vi "Global_Read_INI_Sub_VI_SM.vi"(0 "Config File Path":path) -> (4 "output cluster":T1)   [LabVIEW 2017]
uses:
  <vilib>/Utility/config.llb/Read Key (U32).vi
  <vilib>/Utility/config.llb/Read Key (String).vi
  <vilib>/Utility/config.llb/Read Key (Path).vi
  <vilib>/Utility/config.llb/NI_LVConfig.lvlib
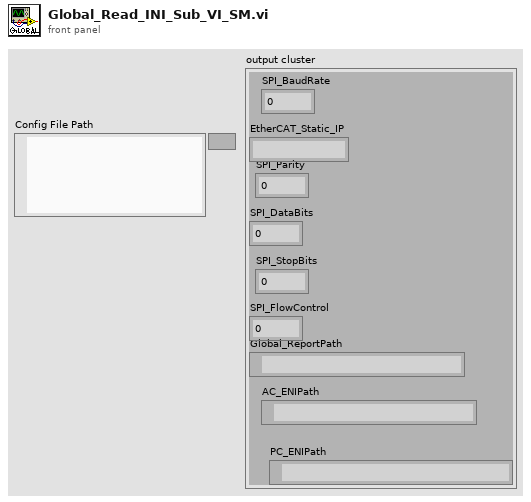
[diagram p1: front panel]
types:
  T1 = cluster{"SPI_BaudRate":u32, "EtherCAT_Static_IP":string, "SPI_Parity":u16, "SPI_DataBits":u16, "SPI_StopBits":u16, "SPI_FlowControl":u16, "Global_ReportPath":path, "AC_ENIPath":path, "PC_ENIPath":path}
  T2 = typedef "NI_LVConfig.lvlib/Config Data RefNum.ctl" = refnum<k1>
  T3 = cluster{u32, "value":string, u16, u16, u16, u16, "value":path, "value":path, "value":path}
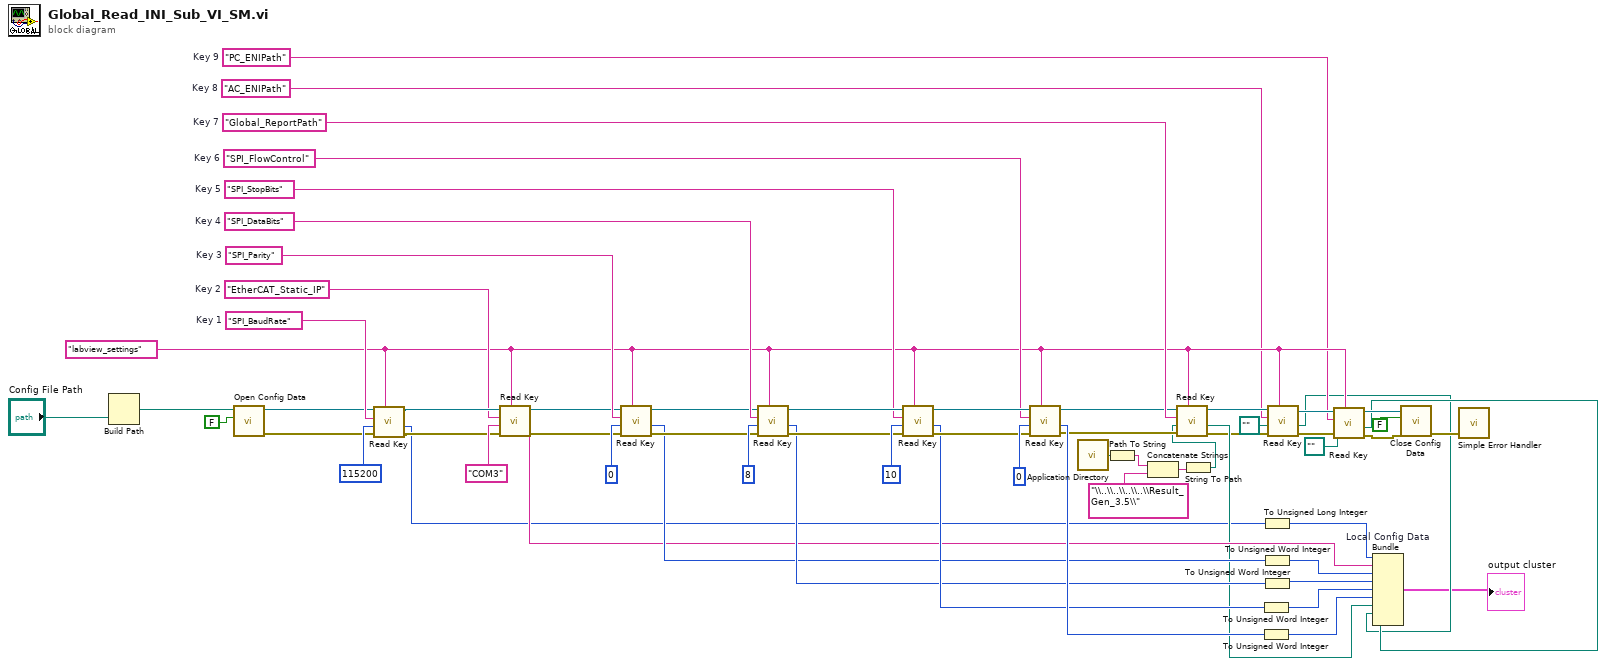
[diagram p0: block diagram]
diagram:
  w6 = "PC_ENIPath"  # Key 9
  w7 = "AC_ENIPath"  # Key 8
  w57 = "Global_ReportPath"  # Key 7
  w53 = "SPI_FlowControl"  # Key 6
  w49 = "SPI_StopBits"  # Key 5
  w47 = "SPI_DataBits"  # Key 4
  w35 = "SPI_Parity"  # Key 3
  w34 = "EtherCAT_Static_IP"  # Key 2
  w40 = "SPI_BaudRate"  # Key 1
  w8 = "labview_settings" ("section")
  n1 = Build Path(name or relative path="Config File Path") -> (appended path=w22:path)  [unwired: 1 in]
  n2 = call <vilib>:"Open Config Data.vi"("create file if necessary (T)"=FALSE ("create file if necessary? (T)"), "configuration file path"=w22) -> ("error out"=w41:errorcluster, "refnum"=w39:T2)  [unwired: 7 in, 1 out]
  n3 = call-poly <vilib>:"Read Key.vi"("section"=w8, "error in (no error)"=w41, "default value"=u32 115200, "key"=w40, "refnum"=w39) -> ("error out"=w42:errorcluster, "value"=w20:u32, "refnum out"=w43:T2)  [unwired: 4 out]
  n4 = call-poly <vilib>:"Read Key.vi"("section"=w8, "error in (no error)"=w42, "default value"="COM3", "key"=w34, "refnum"=w43) -> ("error out"=w33:errorcluster, "value"=w29:string, "refnum out"=w32:T2)  [unwired: 1 in, 3 out]
  n5 = call-poly <vilib>:"Read Key.vi"("section"=w8, "error in (no error)"=w33, "default value"=u32 0, "key"=w35, "refnum"=w32) -> ("error out"=w46:errorcluster, "value"=w44:u32, "refnum out"=w45:T2)  [unwired: 4 out]
  n6 = call-poly <vilib>:"Read Key.vi"("section"=w8, "error in (no error)"=w46, "default value"=u32 8, "key"=w47, "refnum"=w45) -> ("error out"=w51:errorcluster, "value"=w48:u32, "refnum out"=w50:T2)  [unwired: 4 out]
  n7 = call-poly <vilib>:"Read Key.vi"("section"=w8, "error in (no error)"=w51, "default value"=u32 10, "key"=w49, "refnum"=w50) -> ("error out"=w55:errorcluster, "value"=w52:u32, "refnum out"=w54:T2)  [unwired: 4 out]
  n8 = call-poly <vilib>:"Read Key.vi"("section"=w8, "error in (no error)"=w55, "default value"=u32 0, "key"=w53, "refnum"=w54) -> ("error out"=w30:errorcluster, "value"=w56:u32, "refnum out"=w31:T2)  [unwired: 4 out]
  n9 = call <vilib>:"Application Directory.vi"() -> ("Application Directory"=w16:path)
  n10 = Path To String(path=w16) -> (string=w19:string)
  n11 = Concatenate Strings(w19, "\\..\\..\\..\\..\\Result_Gen_3.5\\" ("string")) -> (w17:string)
  n12 = String To Path(string=w17) -> (path=w15:path)
  n13 = call-poly <vilib>:"Read Key.vi"("section"=w8, "error in (no error)"=w30, "default value"=w15, "key"=w57, "refnum"=w31) -> ("error out"=w14:errorcluster, "value"=w24:path, "refnum out"=w13:T2)  [unwired: 1 in, 3 out]
  n14 = To Unsigned Word Integer(number=w52) -> (unsigned 16bit integer=w26:u16)
  n15 = To Unsigned Word Integer(number=w56) -> (unsigned 16bit integer=w25:u16)
  n16 = To Unsigned Long Integer(number=w20) -> (unsigned 32bit integer=w21:u32)
  n17 = To Unsigned Word Integer(number=w44) -> (unsigned 16bit integer=w28:u16)
  n18 = To Unsigned Word Integer(number=w48) -> (unsigned 16bit integer=w27:u16)
  n19 = call-poly <vilib>:"Read Key.vi"("section"=w8, "error in (no error)"=w14, "default value"=path "", "key"=w7, "refnum"=w13) -> ("error out"=w12:errorcluster, "value"=w2:path, "refnum out"=w11:T2)  [unwired: 1 in, 3 out]
  n20 = call-poly <vilib>:"Read Key.vi"("section"=w8, "error in (no error)"=w12, "default value"=path "", "key"=w6, "refnum"=w11) -> ("error out"=w9:errorcluster, "value"=w5:path, "refnum out"=w10:T2)  [unwired: 1 in, 3 out]
  n21 = Bundle "Local Config Data"(w21, "value"=w29, w28, w27, w26, w25, "value"=w24, "value"=w2, "value"=w5) -> (→"output cluster":T3)  [unwired: 1 in]
  n22 = call <vilib>:"Close Config Data.vi"("error in (no error)"=w9, "write file if changed (T)"=FALSE ("write configuration file? (T)"), "refnum"=w10) -> ("error out"=w38:errorcluster)  [unwired: 8 out]
  n23 = call <vilib>:"Simple Error Handler.vi"("error in (no error)"=w38) -> ()  [unwired: 1 in, 8 out]
